vi "Objects bottom cords.vi"(2 "error in (no error)":errorcluster, 3 "Image":T4) -> (0 "error out":errorcluster, 1 "Objects bottom cords":T3(array[cluster]))   [LabVIEW 2009, in "ImageAnalysis.lvlib"]
doc: "Inputs:\nA binary image where white spotts are objects to detect.\n\nOutput:\nA 1-D array with a cluster element per detected object. Each cluster contains a 1-D array with the detected bottom points of the object."
uses:
  ImageAnalysis.lvlib
  <vilib>/vision/Image Controls.llb/IMAQ Image.ctl
  <vilib>/Analysis/Matrix/Numeric/Conversions/Array To Matrix - RA2.vi
  <vilib>/vision/NI_Vision_Development_Module.lvlib
  <vilib>/Analysis/Matrix/NI_Matrix.lvlib
panel:
  in  "Object":T1
  out "Rectangle":T2 {"Rotation" format="%.2f"; "Left" scale=0.0..1024.0; "Right" scale=0.0..1024.0; "Bottom" scale=1024.0..0.0; "Top" scale=1024.0..0.0}
  in  "Rectangle cluster":T2 {"Rotation" min=-90.0 max=90.0 step=1.0 format="%.2f"; "Left" scale=0.0..1024.0; "Right" scale=0.0..1024.0; "Bottom" scale=1024.0..0.0; "Top" scale=1024.0..0.0}
  # "Excecution time for this node is approx: 350 ms"
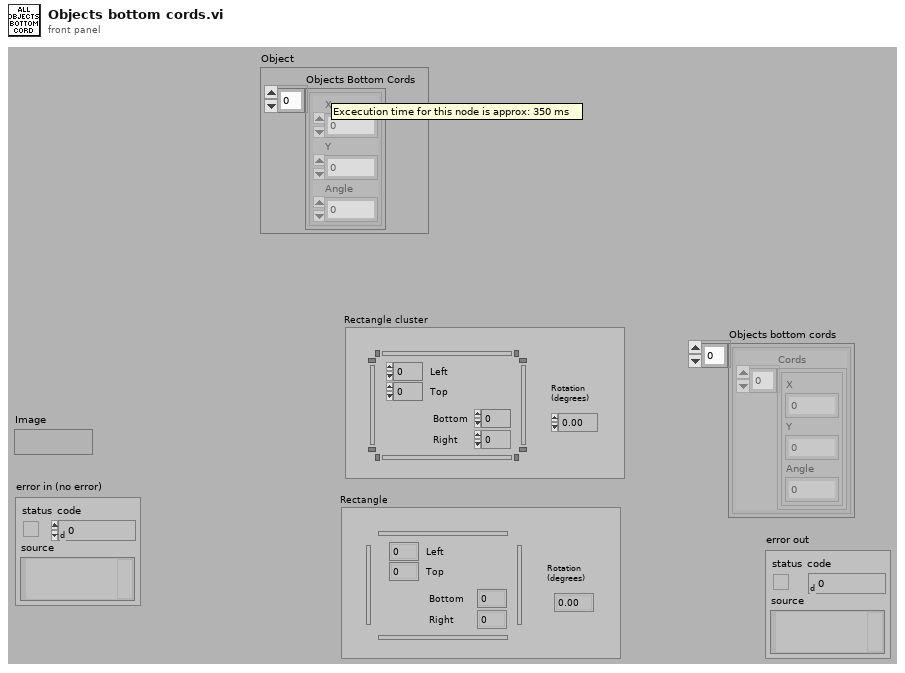
[diagram p1: front panel]
types:
  T1 = cluster{"Objects Bottom Cords":cluster{"X":dbl, "Y":dbl, "Angle":dbl}[]}
  T2 = typedef "IMAQ Rectangle" = cluster{"Left":i32, "Top":i32, "Right":i32, "Bottom":i32, "Rotation":dbl}
  T3 = cluster{"Cords":cluster{"X":dbl, "Y":dbl, "Angle":dbl}[]}[]
  T4 = typedef "IMAQ Image.ctl" = refnum<image>
  T5 = typedef "Particle Parameters" = i32
  T6 = typedef "Image Type" = u32
  T7 = cluster{"Objects Bottom Cords":cluster{"X":dbl, "Y":dbl, "Angle":dbl}[]}[]
  T8 = typedef "NI_Matrix.lvlib/RealMatrix.ctl" = dbl[][]
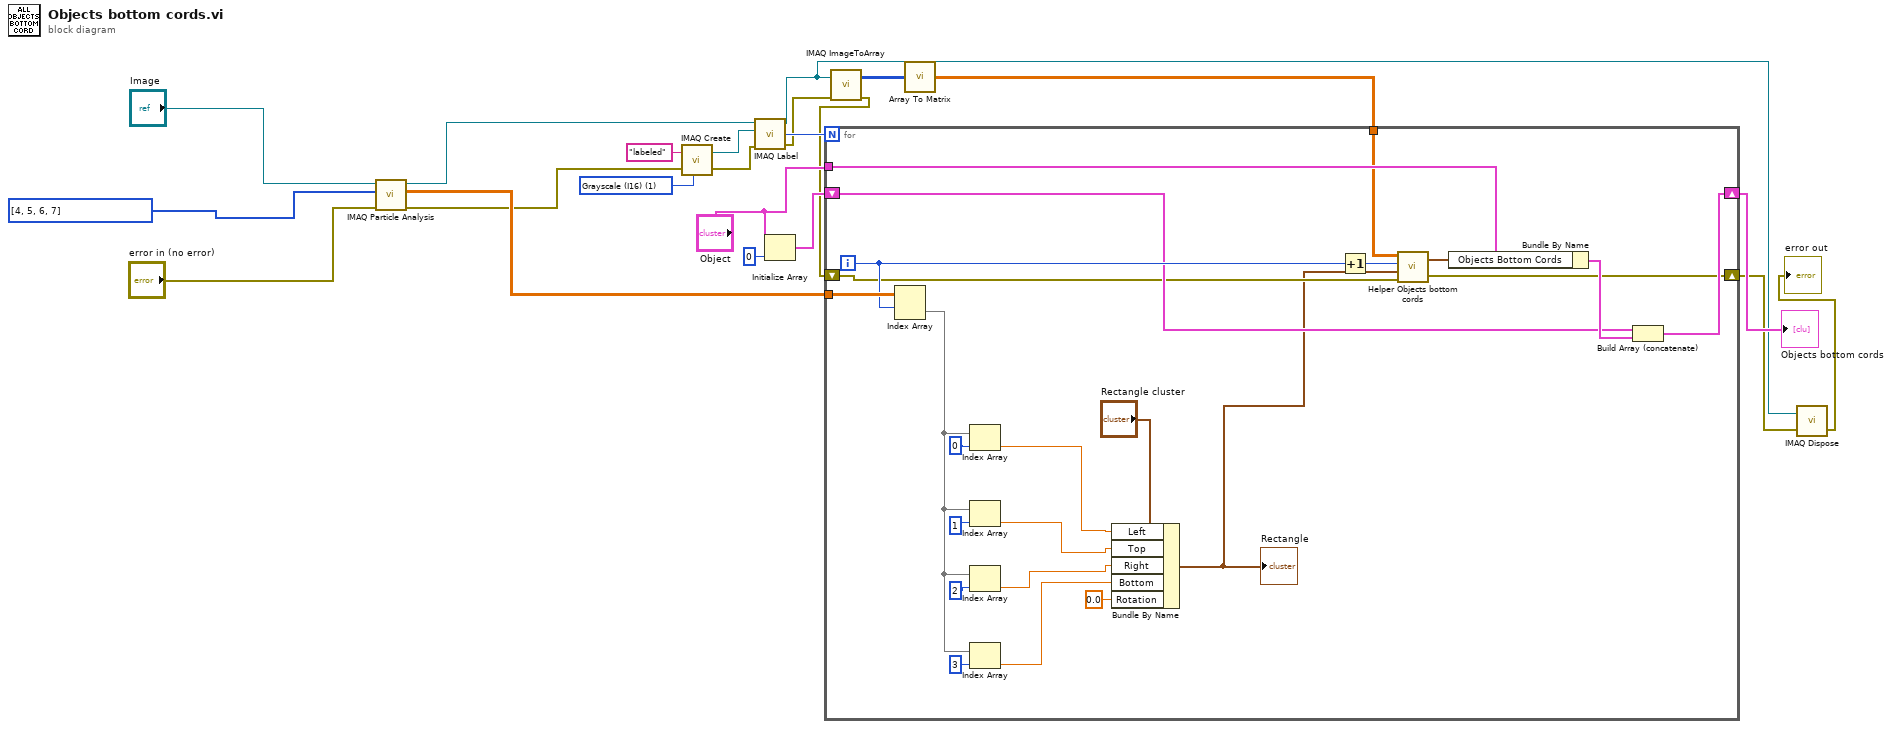
[diagram p0: block diagram]
diagram:
  w9 = T5[] [4, 5, 6, 7] items=["Center of Mass X", "Center of Mass Y", "First Pixel X", "First Pixel Y", "Bounding Rect Left", "Bounding Rect Top", "Bounding Rect Right", "Bounding Rect Bottom", "Max Feret Diameter Start X", "Max Feret Diameter Start Y", "Max Feret Diameter End X", "Max Feret Diameter End Y", "Max Horiz. Segment Length Left", "Max Horiz. Segment Length Right", "Max Horiz. Segment Length Row", "-", "Bounding Rect Width", "Bounding Rect Height", "Bounding Rect Diagonal", "Perimeter", "Convex Hull Perimeter", "Holes' Perimeter", "Max Feret Diameter", "Equivalent Ellipse Major Axis", "Equivalent Ellipse Minor Axis", "Equivalent Ellipse Minor Axis (Feret)", "Equivalent Rect Long Side", "Equivalent Rect Short Side", "Equivalent Rect Diagonal", "Equivalent Rect Short Side (Feret)", "Average Horiz. Segment Length", "Average Vert. Segment Length", "Hydraulic Radius", "Waddel Disk Diameter", "-", "Area", "Holes' Area", "Particle & Holes' Area", "Convex Hull Area", "Image Area", "-", "Number of Holes", "Number of Horiz. Segments", "Number of Vert. Segments", "-", "Orientation", "Max Feret Diameter Orientation", "-", "% Area/Image Area", "% Area/(Particle & Holes' Area)", "Ratio of Equivalent Ellipse Axes", "Ratio of Equivalent Rect Sides", "-", "Elongation Factor", "Compactness Factor", "Heywood Circularity Factor", "Type Factor", "-", "Sum X", "Sum Y", "Sum XX", "Sum XY", "Sum YY", "Sum XXX", "Sum XXY", "Sum XYY", "Sum YYY", "-", "Moment of Inertia XX", "Moment of Inertia XY", "Moment of Inertia YY", "Moment of Inertia XXX", "Moment of Inertia XXY", "Moment of Inertia XYY", "Moment of Inertia YYY", "Norm. Moment of Inertia XX", "Norm. Moment of Inertia XY", "Norm. Moment of Inertia YY", "Norm. Moment of Inertia XXX", "Norm. Moment of Inertia XXY", "Norm. Moment of Inertia XYY", "Norm. Moment of Inertia YYY", "Hu Moment 1", "Hu Moment 2", "Hu Moment 3", "Hu Moment 4", "Hu Moment 5", "Hu Moment 6", "Hu Moment 7"] ("Pixel Measurements")
  w18 = T6 1 items=["Grayscale (U8)", "Grayscale (I16)", "Grayscale (SGL)", "Complex (CSG)", "RGB (U32)", "HSL (U32)", "RGB (U64)", "Grayscale (U16)"] ("Image Type")
  n1 = call "IMAQ Particle Analysis"("error in (no error)"="error in (no error)", "Pixel Measurements"=w9, "Image"="Image") -> ("error out"=w8:errorcluster, "Particle Measurements (Pixels)"=w14:dbl[][], "Image Out (duplicate)"=w20:T4)  [unwired: 3 in, 3 out]
  n2 = call "IMAQ Create"("Image Name"="labeled", "Image Type"=w18, "error in (no error)"=w8) -> ("New Image"=w17:T4, "error out"=w7:errorcluster)  [unwired: 2 in]
  n3 = call "IMAQ Label"("error in (no error)"=w7, "Image Dst"=w17, "Image Src"=w20) -> ("error out"=w2:errorcluster, "Number of Particles"=w15:i32, "Image Dst Out"=w5:T4)  [unwired: 1 in]
  n4 = Initialize Array("Object", 0 ("dimension size")) -> (w11:T7)
  n5 = call "IMAQ ImageToArray"("error in (no error)"=w2, "Image"=w5) -> ("error out"=w1:errorcluster, "Image Pixels (I16)"=w16:i16[][])  [unwired: 2 in, 3 out]
  n6 = call-poly <vilib>:"Array To Matrix.vi"("Real 2D Array"=w16) -> ("Real Matrix"=w13:T8)
  n7 = for {
    N: w15 -> [_]
    tunnel: w14 -> [w32]
    tunnel: w13 -> [w25]
    shift-right: [w29] -> w6
    shift-left: w11 -> [w30]
    tunnel: "Object" -> [w28]
    shift-right: [w26] -> w4
    shift-left: w1 -> [w27]
    i -> [w31]
    n8 = Index Array(array=w32, index (row)=w31) -> (element=w33:dbl[])  [unwired: 1 in]
    n9 = Index Array(array=w33, index=0) -> (element=w34:dbl)
    n10 = Index Array(array=w33, index=1) -> (element=w35:dbl)
    n11 = Index Array(array=w33, index=2) -> (element=w36:dbl)
    n12 = Index Array(array=w33, index=3) -> (element=w37:dbl)
    n13 = Bundle By Name(cluster="Rectangle cluster", "Left"=w34, "Top"=w35, "Right"=w36, "Bottom"=w37, "Rotation"=0.0) -> (w24:T2)
    "Rectangle" <- w24
    n14 = Increment(x=w31) -> (x+1=w45:i32)
    n15 = call "Helper Objects bottom cords.vi"("error in (no error)"=w27, "Rectangle"=w24, "Object color"=w45, "Image matrix"=w25) -> ("error out"=w26:errorcluster, "Objects Bottom Cords"=w23:cluster{"X":dbl, "Y":dbl, "Angle":dbl}[])
    n16 = Bundle By Name(cluster=w28, "Objects Bottom Cords"=w23) -> (w44:T1)
    n17 = Build Array (concatenate)(w30, w44) -> (w29:T7)
  }
  "Objects bottom cords" <- w6
  n18 = call "IMAQ Dispose"("Image"=w5, "error in (no error)"=w4) -> ("error out"=→"error out":errorcluster)  [unwired: 4 in]
